vi "Autosize Table Cells.vi"(9 "Table Data in":string[][](array[string]), 10 "Column to Autosize":i32, 11 "Table Ref in":refnum<vi>) -> ()   [LabVIEW 2019]
uses:
  <vilib>/Utility/miscctls.llb/LVRowAndColumnTypeDef.ctl
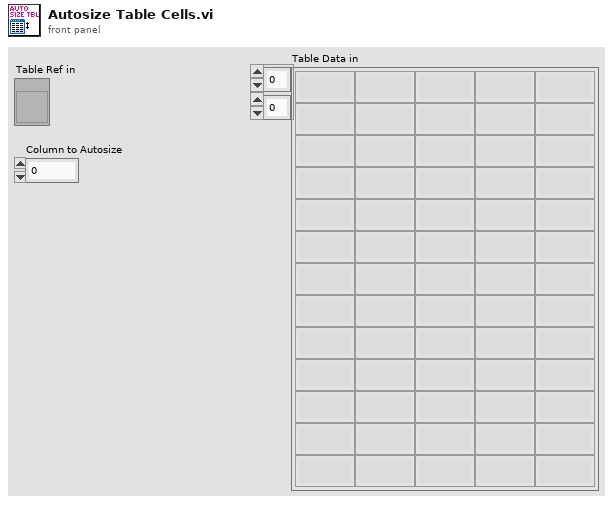
[diagram p1: front panel]
types:
  T1 = typedef "LVRowAndColumnTypeDef.ctl" = cluster{"Row":i32, "Column":i32}
  T2 = cluster{"left":i16, "top":i16, "right":i16, "bottom":i16}
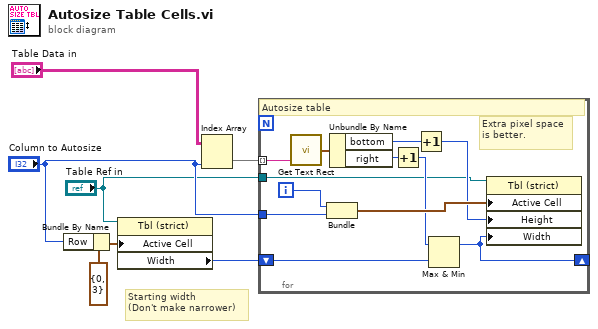
[diagram p0: block diagram]
diagram:
  # "Starting width\n(Don't make narrower)"
  n1 = Bundle By Name(cluster=T1 {"Row"=0, "Column"=3} ("Active Cell:Active Cell"), "Row"="Column to Autosize") -> (w6:T1)
  n2 = property on="Property Node" class="Tbl (strict)"(reference="Table Ref in", "Active Cell"=w6) -> ("Width"=w4:u32)  [unwired: 1 in, 2 out]
  n3 = Index Array(array="Table Data in", index (col)="Column to Autosize") -> (element=w3:string[])  [unwired: 1 in]
  n4 = for {
    tunnel: w3 -> [w19] mode=indexing
    tunnel: "Column to Autosize" -> [w16]
    shift-right: [w13] -> _
    shift-left: w4 -> [w14]
    tunnel: "Table Ref in" -> [w8]
    i -> [w17]
    # "Extra pixel space is better."
    # "Autosize table"
    n5 = call <vilib>:"Get Text Rect.vi"("text"=w19) -> ("rect"=w15:T2)  [unwired: 8 in]
    n6 = Bundle(w17, "Column to Autosize"=w16) -> (w18:cluster{i32, "Column to Autosize":i32})  [unwired: 1 in]
    n7 = Unbundle By Name(w15) -> ("bottom"=w10:i16, "right"=w12:i16)
    n8 = Increment(x=w12) -> (x+1=w11:i16)
    n9 = Increment(x=w10) -> (x+1=w9:i16)
    n10 = Max & Min(x=w11, y=w14) -> (max(x,y)=w13:u32)  [unwired: 1 out]
    n11 = property on="Property Node" class="Tbl (strict)"(reference=w8, "Active Cell"=w18, "Height"=w9, "Width"=w13) -> ()  [unwired: 1 in, 2 out]
  }
